vi "00 - Calling Python Simple.vi"() -> ()   [LabVIEW 2026]
uses:
  <vilib>/Utility/sysdir.llb/System Directory Type.ctl
panel:
  out "Intensity Graph":dbl[][](graph)
  in  "Colormap to Extract":string="viridis"
  out "return value":cluster{"R":dbl, "G":dbl, "B":dbl, "A":dbl}[](array[cluster])
  out "Colormap Names":string[](array[string])
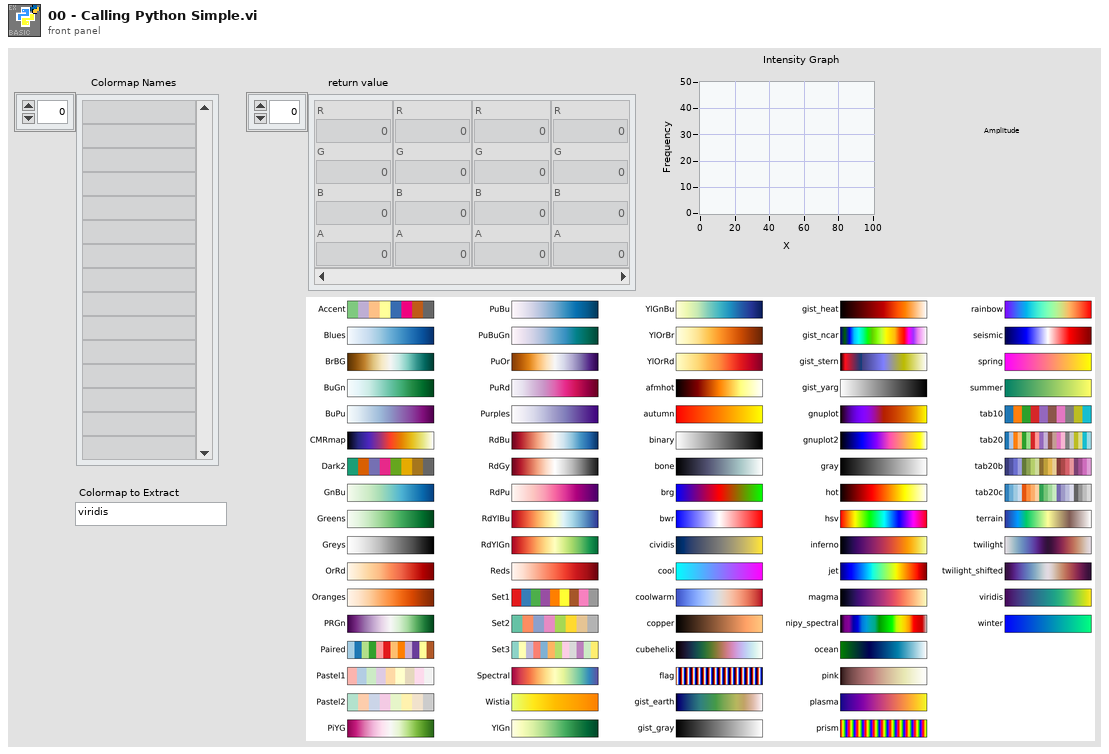
[diagram p1: front panel]
types:
  T1 = typedef "System Directory Type.ctl" = i32
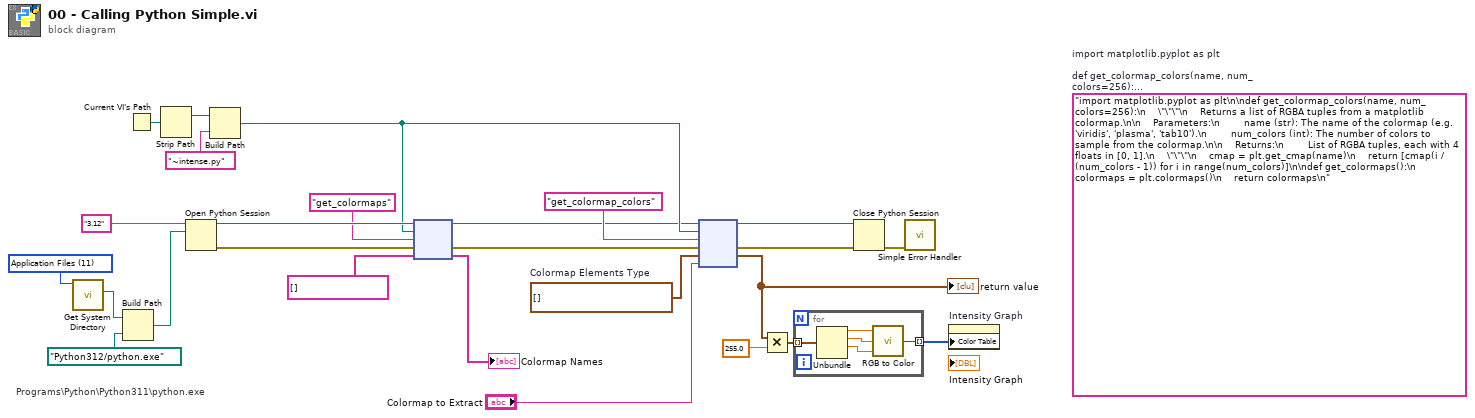
[diagram p0: block diagram]
diagram:
  w8 = T1 11 items=["User Home"=0, "User Desktop"=1, "User Documents"=2, "User Application Data"=3, "User Preferences"=4, "User Temporary"=5, "Public Documents"=6, "Public Application Data"=7, "Public Preferences"=8, "Public Cache"=13, "System Core Libraries"=9, "System Installed Libraries"=10, "Application Files"=11, "Boot Volume Root"=12] ("system directory type")
  w26 = cluster{"R":dbl, "G":dbl, "B":dbl, "A":dbl}[] []  # Colormap Elements Type
  (unwired) "import matplotlib.pyplot as plt\n\ndef get_colormap_colors(name, num_colors=256):\n    \"\"\"\n    Returns a list of RGBA tuples from a matplotlib colormap.\n\n    Parameters:\n        name (str): The name of the colormap (e.g. 'viridis', 'plasma', 'tab10').\n        num_colors (int): The number of colors to sample from the colormap.\n\n    Returns:\n        List of RGBA tuples, each with 4 floats in [0, 1].\n    \"\"\"\n    cmap = plt.get_cmap(name)\n    return [cmap(i / (num_colors - 1)) for i in range(num_colors)]\n\ndef get_colormaps():\n    colormaps = plt.colormaps()\n    return colormaps\n"  # import matplotlib.pyplot as plt  def get_colormap_colors(name, num_colors=256):     """     Returns a list of RGBA tuples from a matplotlib colormap.      Parameters:         name (str): The name of the colormap (e.g. 'viridis', 'plasma', 'tab10').         num_colors (int): The number of colors to sample from the colormap.      Returns:         List of RGBA tuples, each with 4 floats in [0, 1].     """     cmap = plt.get_cmap(name)     return [cmap(i / (num_colors - 1)) for i in range(num_colors)]  def get_colormaps():     colormaps = plt.colormaps()     return colormaps
  # "Programs\\Python\\Python311\\python.exe"
  n1 = call <vilib>:"Get System Directory.vi"("system directory type"=w8) -> ("system directory"=w7:path)  [unwired: 10 in]
  n2 = Build Path(base path=w7, name or relative path=path "Python312/python.exe") -> (appended path=w6:path)
  n3 = Current VI's Path() -> (path=w17:path)
  n4 = Strip Path(path=w17) -> (stripped path=w18:path)  [unwired: 1 out]
  n5 = Open Python Session(python version="3.12" ("Python version"), python path=w6) -> (session out=w24:refnum<k35>, error out=w25:errorcluster)  [unwired: 1 in]
  n6 = Build Path(base path=w18, name or relative path="~intense.py" ("function name")) -> (appended path=w14:path)
  n7 = node(w24, w14, "get_colormaps" ("function name"), w25, string[] [] ("function name")) -> (w13:refnum<k35>, w12:errorcluster, →"Colormap Names":string[])  [unwired: 2 out]
  n8 = node(w13, w14, "get_colormap_colors" ("function name"), w12, w26, "Colormap to Extract") -> (w10:refnum<k35>, w11:errorcluster, w4:cluster{"R":dbl, "G":dbl, "B":dbl, "A":dbl}[])  [unwired: 1 in, 2 out]
  "return value" <- w4
  n9 = Multiply(x=w4, y=255.0 ("A")) -> (x*y=w3:cluster{"R":dbl, "G":dbl, "B":dbl, "A":dbl}[])
  n10 = for {
    tunnel: w3 -> [w31] mode=indexing
    tunnel: [w27] -> w1 mode=indexing
    n11 = Unbundle(w31) -> ("R"=w30:dbl, "G"=w29:dbl, "B"=w28:dbl)  [unwired: 1 out]
    n12 = call <vilib>:"RGB to Color.vi"("B"=w28, "G"=w29, "R"=w30) -> ("Color"=w27:u32)
  }
  n13 = Close Python Session(session in=w10, error in=w11) -> (11:w19:errorcluster)
  n14 = call <vilib>:"Simple Error Handler.vi"("error in (no error)"=w19) -> ()  [unwired: 4 in, 5 out]
  n15 = property on="Intensity Graph" class="IntGraph (strict)"("Color Table"=w1) -> ()  [unwired: 2 in, 2 out]
